vi "23384_Davis_Poku_Amankwa_Amankwa.DavisPoku.MNE1201.1.4_348251_856158138.vi"() -> ()   [LabVIEW 2018]
panel:
  out "Sine of Angle":dbl
  in  "Angle in degrees":dbl
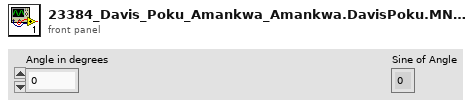
[diagram p1: front panel]
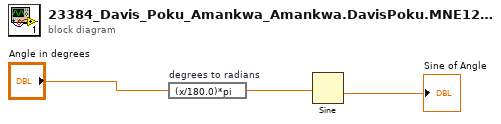
[diagram p0: block diagram]
diagram:
  n1 = expression code="(x/180.0)*pi" "degrees to radians"("Angle in degrees") -> (w2:dbl)
  n2 = Sine(x=w2) -> (sin(x)=→"Sine of Angle":dbl)
